vi "Update ARINC.vi"(8 "error in":errorcluster, 11 "ARINC":sgl[](array[numeric])) -> (0 "error out":errorcluster)   [LabVIEW 2018, in "UDP Writer.lvlib"]
doc: "This subVI enqueues the named action in to the communications queue along with the input data."
uses:
  UDP Writer.lvlib
  Private Controls/Module Data.ctl
  Private Controls/Module Action.ctl
  370fc90e-dbb7-4a90-8f75-05d8fabf3903.vi
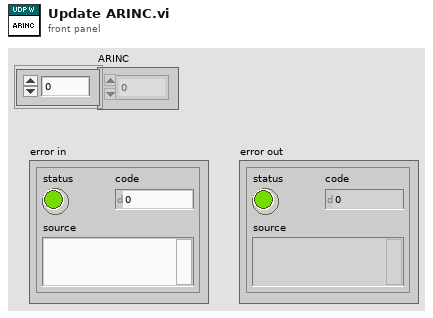
[diagram p1: front panel]
types:
  T1 = typedef "UDP Writer.lvlib/Module Data.ctl" = cluster{"Data":variant, "Action":T2}
  T2 = typedef "UDP Writer.lvlib/Module Action.ctl" = enum16{"Init", "Update ARINC", "Update Waterfall", "Update RPMs", "Update Temps", "Update Modbus", "Update AI", "Update Vibs", "Write", "Error"}
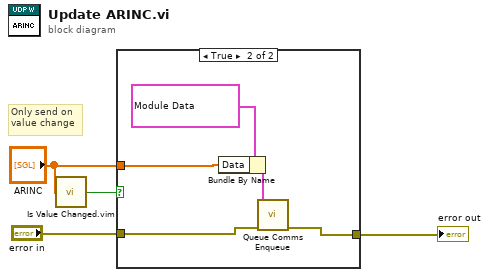
[diagram p0: block diagram]
diagram:
  # "Only send on\nvalue change"
  n1 = call "Is Value Changed.vim"("value"="ARINC") -> ("changed or first call?"=w1:bool)
  n2 = case shown="True" w1 {
    tunnel: [w5 w10] -> w4
    tunnel: "error in" -> [w5 w9]
    tunnel: "ARINC" -> [_ w6]
    frame False {
    }
    frame True {
      n3 = Bundle By Name(cluster=T1 {"Data"=variant, "Action"=enum."Update ARINC"} ("element"), "Data"=w6) -> (w7:T1)
      n4 = call "Queue Comms Enqueue.vi"("error in (no error)"=w9, "element"=w7) -> ("error out"=w10:errorcluster)  [unwired: 9 in]
    }
  }
  "error out" <- w4
